vi "Novo_tempo_obs_inicial.vi"(9 "TS":dbl, 10 "RA":dbl, 11 "DEC":dbl) -> (2 "TO horas":dbl, 3 "TO rad":dbl)   [LabVIEW 2018]
uses:
  Global_Telescopio.vi
panel:
  out "AH norm":dbl
  out "Numeric":i32
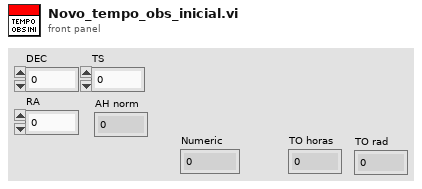
[diagram p1: front panel]
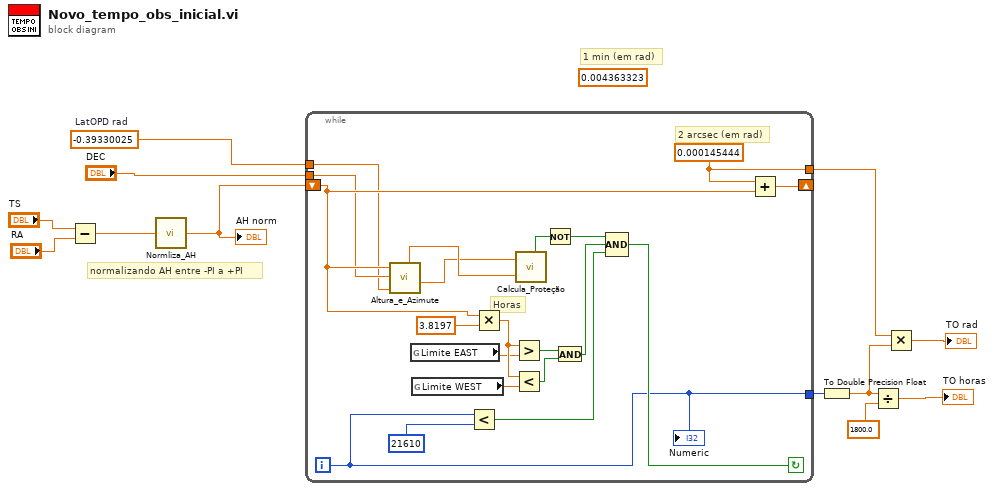
[diagram p0: block diagram]
diagram:
  w6 = -0.39330025  # LatOPD rad
  (unwired) 0.004363323
  # "normalizando AH entre -PI a +PI"
  # "1 min (em rad)"
  n1 = Subtract(x="TS", y="RA") -> (x-y=w2:dbl)
  n2 = call "Normliza_AH.vi"("PosAH"=w2) -> ("Numeric"=w1:dbl)
  "AH norm" <- w1
  n3 = while {
    tunnel: w6 -> [w15]
    tunnel: "DEC" -> [w16]
    shift-right: [w22] -> _
    shift-left: w1 -> [w17]
    tunnel: [w20] -> w12
    tunnel: [w21] -> w9
    i -> [w20]
    stop <- w23 continue-if-true
    w21 = 0.000145444
    # "2 arcsec (em rad)"
    # "Horas"
    n4 = call "Altura_e_Azimute.vi"("LAT rad"=w15, "DEC rad"=w16, "AH rad"=w17) -> ("AZIMUTE rad"=w13:dbl, "ANG. ZENITAL rad"=w14:dbl)  [unwired: 4 out]
    n5 = global read "Global_Telescopio.vi" "Limite EAST"() -> (w26:dbl)
    n6 = global read "Global_Telescopio.vi" "Limite WEST"() -> (w27:dbl)
    n7 = Less?(x=w20, y=21610) -> (x < y?=w18:bool)
    n8 = Multiply(x=w17, y=3.8197) -> (x*y=w30:dbl)
    n9 = Greater?(x=w30, y=w26) -> (0:w29:bool)
    n10 = Less?(x=w30, y=w27) -> (x < y?=w25:bool)
    n11 = call "Calcula_Proteção.vi"("Zenital angle rad"=w14, "Azimute rad"=w13) -> ("Prot Zmax"=w32:bool)  [unwired: 4 out]
    n12 = Not(x=w32) -> (.not. x?=w28:bool)
    n13 = And(x=w29, y=w25) -> (x .and. y?=w24:bool)
    n14 = Compound Arithmetic op=AND(w28, w24, w18) -> (w23:bool)
    n15 = Add(x=w21, y=w17) -> (x+y=w22:dbl)
    "Numeric" <- w20
  }
  n16 = To Double Precision Float(number=w12) -> (double precision float=w8:dbl)
  n17 = Divide(x=w8, y=1800.0) -> (x/y=→"TO horas":dbl)
  n18 = Multiply(x=w9, y=w8) -> (x*y=→"TO rad":dbl)
